vi "DPT MA Scale Corrections.vi"(1 "RMC Calc Inputs":T1, 2 "Enable":bool=TRUE, 3 "MA Filter Size":i32=60, 8 "Reset":bool) -> (14 "RMC_Sm":dbl, 15 "RMC":dbl format="%.2f", 16 "Raw Weight":dbl format="%.2f", 17 "Corrected Weight":dbl format="%.2f", 18 "Wcomp":dbl, 19 "Wbouy":dbl)   [LabVIEW 2016]
uses:
  Type Definitions/RMC Calc Inputs.ctl
  <vilib>/Analysis/baseanly.llb/Mean (DBL).vi
  <vilib>/Analysis/NI_AALBase.lvlib
panel:
  out "appended array":dbl[](array[numeric])
  out "Smoothed Weight":dbl
  out "Count":dbl
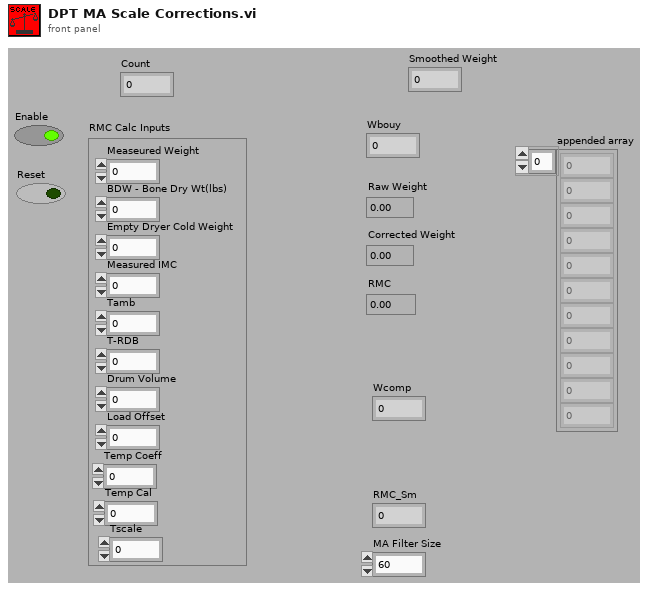
[diagram p1: front panel]
types:
  T1 = typedef "RMC Calc Inputs.ctl" = cluster{"Measeured Weight":dbl, "BDW - Bone Dry Wt(lbs)":dbl, "Empty Dryer Cold Weight":dbl, "Measured IMC":dbl, "Tamb":dbl, "T-RDB":dbl, "Drum Volume":dbl, "Load Offset":dbl, "Temp Coeff":dbl, "Temp Cal":dbl, "Tscale":dbl}
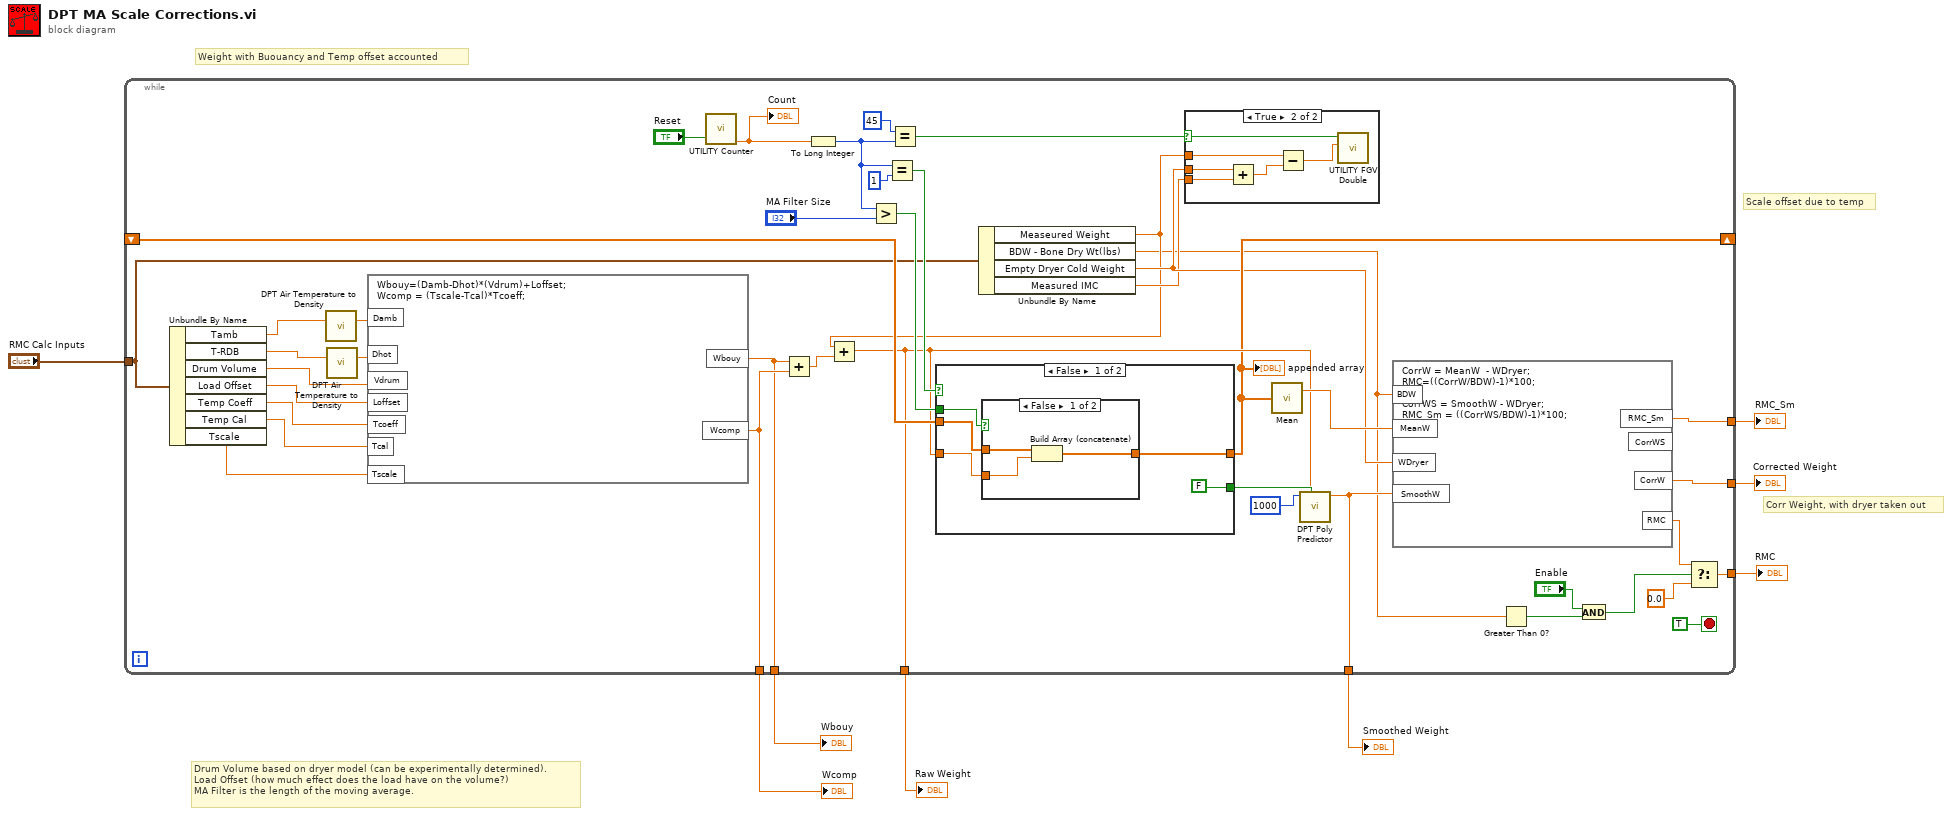
[diagram p0: block diagram]
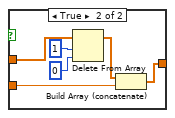
[diagram p3: hidden frame]
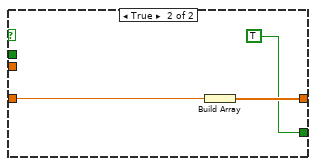
[diagram p4: hidden frame]
diagram:
  # "Corr Weight, with dryer taken out"
  # "Weight with Buouancy and Temp offset accounted"
  # "Scale offset due to temp"
  # "Drum Volume based on dryer model (can be experimentally determined).\nLoad Offset (how much effect does the load have on the volume?)\nMA Filter is the length of the moving average."
  n1 = while {
    tunnel: "RMC Calc Inputs" -> [w13]
    shift-right: [w17] -> _
    shift-left: _ -> [w49]
    tunnel: [w32] -> w8
    tunnel: [w19] -> w7
    tunnel: [w15] -> w6
    tunnel: [w30] -> w4
    tunnel: [w16] -> w1
    tunnel: [w24] -> w3
    tunnel: [w22] -> w2
    stop <- TRUE stop-if-true
    n2 = Unbundle By Name(w13) -> ("Tamb"=w43:dbl, "T-RDB"=w42:dbl, "Drum Volume"=w40:dbl, "Load Offset"=w41:dbl, "Temp Coeff"=w37:dbl, "Temp Cal"=w36:dbl, "Tscale"=w34:dbl)
    n3 = call "DPT Air Temperature to Density.vi"("Temp(F)"=w43) -> ("Density (lb/ft3)"=w39:dbl)  [unwired: 14 in]
    n4 = call "DPT Air Temperature to Density.vi"("Temp(F)"=w42) -> ("Density (lb/ft3)"=w38:dbl)  [unwired: 14 in]
    n5 = formula code="Wbouy=(Damb-Dhot)*(Vdrum)+Loffset;\nWcomp = (Tscale-Tcal)*Tcoeff;"("Damb"=w39, "Dhot"=w38, "Vdrum"=w40, "Loffset"=w41, "Tscale"=w34, "Tcal"=w36, "Tcoeff"=w37) -> ("Wbouy"=w16:dbl, "Wcomp"=w30:dbl)
    n6 = call "UTILITY Counter.vi"("Reset"="Reset") -> ("Count"=w27:dbl)  [unwired: 10 in]
    "Count" <- w27
    n7 = Add(x=w16, y=w30) -> (x+y=w35:dbl)
    n8 = To Long Integer(number=w27) -> (32bit integer=w20:i32)
    n9 = Greater?(x=w20, y="MA Filter Size") -> (0:w44:bool)
    n10 = Equal?(x=w20, y=1) -> (x = y?=w47:bool)
    n11 = Equal?(x=45 ("y"), y=w20) -> (x = y?=w18:bool)
    n12 = Unbundle By Name(w13) -> ("Measeured Weight"=w10:dbl, "BDW - Bone Dry Wt(lbs)"=w9:dbl, "Empty Dryer Cold Weight"=w12:dbl, "Measured IMC"=w11:dbl)
    n13 = Add(x=w10, y=w35) -> (x+y=w19:dbl)
    n14 = case shown="False" w47 {
      tunnel: w19 -> [w61 w73]
      tunnel: w49 -> [w60 _]
      tunnel: [w59 w72] -> w17
      tunnel: w44 -> [w58 _]
      tunnel: [FALSE TRUE] -> w25
      frame False {
        n15 = case shown="False" w58 {
          tunnel: [w64 w65] -> w59
          tunnel: w61 -> [w63 w66]
          tunnel: w60 -> [w62 w70]
          frame False {
            n16 = Build Array (concatenate)(w62, w63) -> (w64:dbl[])
          }
          frame True {
            n17 = Delete From Array(array=w70, length=1, index=0) -> (array with subset deleted=w67:dbl[])  [unwired: 1 out]
            n18 = Build Array (concatenate)(w67, w66) -> (w65:dbl[])
          }
        }
      }
      frame True {
        n19 = Build Array(w73) -> (w72:dbl[])
      }
    }
    "appended array" <- w17
    n20 = case shown="True" w18 {
      selector: w18 -> [_ w56]
      tunnel: w10 -> [_ w55]
      tunnel: w11 -> [_ w54]
      tunnel: w12 -> [_ w53]
      frame False {
      }
      frame True {
        n21 = Add(x=w53, y=w54) -> (x+y=w52:dbl)
        n22 = Subtract(x=w55, y=w52) -> (x-y=w51:dbl)
        n23 = call "UTILITY FGV Double.vi"("Value In"=w51, "Set?"=w56) -> ()  [unwired: 9 in, 1 out]
      }
    }
    n24 = call-poly <vilib>:"Mean.vi"("X"=w17) -> ("mean"=w48:dbl)  [unwired: 1 out]
    n25 = call "DPT Poly Predictor.vi"("Initialize"=w25, "Weight"=w19, "Number of Values to Smooth"=1000) -> ("Smoothed Value"=w24:dbl)  [unwired: 8 in]
    n26 = formula code="CorrW = MeanW  - WDryer;\nRMC=((CorrW/BDW)-1)*100;\n\nCorrWS = SmoothW - WDryer;\nRMC_Sm = ((CorrWS/BDW)-1)*100;"("BDW"=w9, "MeanW"=w48, "WDryer"=w12, "SmoothW"=w24) -> ("CorrW"=w15:dbl, "RMC"=w33:dbl, "RMC_Sm"=w22:dbl)  [unwired: 1 out]
    n27 = Greater Than 0?(x=w9) -> (x > 0?=w29:bool)
    n28 = And(x="Enable", y=w29) -> (x .and. y?=w28:bool)
    n29 = Select(t=w33, s=w28, f=0.0) -> (s? t:f=w32:dbl)
  }
  "RMC" <- w8
  "Corrected Weight" <- w6
  "Raw Weight" <- w7
  "Wcomp" <- w4
  "Wbouy" <- w1
  "Smoothed Weight" <- w3
  "RMC_Sm" <- w2
